vi "Read Command Status Ref.vi"(8 "error in (no error)":errorcluster, 11 "Command in":refnum<class "Command.lvclass">) -> (0 "error out":errorcluster, 2 "Command Status Ref":refnum<vi>, 3 "Command out":refnum<class "Command.lvclass">)   [LabVIEW 2013, in "Robot Actors.lvlib" / "Command.lvlib" / "Command.lvclass"]
uses:
  Command.lvclass
  Command Status.ctl
  Command States.ctl
  Command.lvclass/Command.ctl
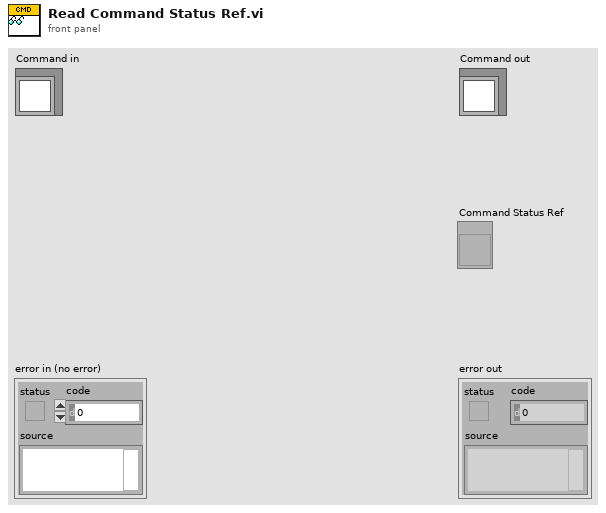
[diagram p1: front panel]
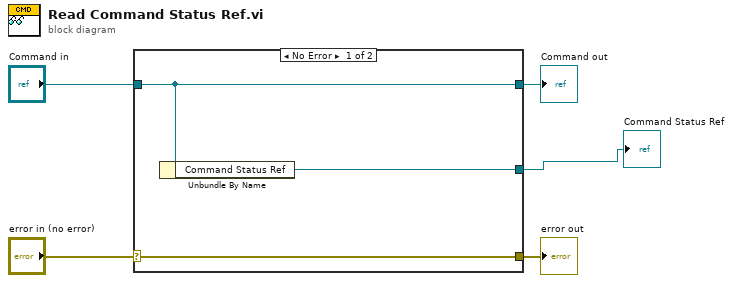
[diagram p0: block diagram]
diagram:
  n1 = case shown="No Error" "error in (no error)" {
    selector: "error in (no error)" -> [w8 w9]
    tunnel: [w8 w9] -> w4
    tunnel: [w7 w10] -> w2
    tunnel: "Command in" -> [w7 w10]
    tunnel: [w6 _] -> w1
    frame No Error {
      n2 = Unbundle By Name(w7) -> ("Command Status Ref"=w6:refnum<vi>)
    }
    frame Error {
    }
  }
  "error out" <- w4
  "Command out" <- w2
  "Command Status Ref" <- w1
